vi "auto_transfer_output_dimension_withburnin.vi"() -> ()   [LabVIEW 2018]
panel:
  in  "Thickness (nm)":string
  in  "Dimension(No.:1-8)":fxp<+,8,8>=1.0 caption="Dimension"
  in  "Email on completion?":bool
  in  "Email recipient":string="rgiri@uw.edu"
  in  "Subject":string="OECT Scans Done"
  in  "Message":string="Hi Raj"
  out "Current Scan #":dbl
  out "Current V_G":dbl
  in  "Transfer Curve Controls":T1={"V_G Start"=-0.85, "V_G Finish"=0.0, "V_G Step Size"=0.025, "Software Averages"=5, "Delay between \naverages (ms)"=200.0, "Preread delay (ms)"=5000.0, "First bias settle (ms)"=2000.0, "V_DS"=-0.6, "Current Compliance\nLimit 237 (A)"=0.1, "Keithley 237 GPIB address"="17", "Current Compliance\nLimit (A) Ke2400"=1.0, "VISA resource name "="GPIB0::24::INSTR", "Number of Transfer Curves"=1.0, "Voltage Compliance Limit 237 (V)"=10.0} {"Voltage Compliance Limit 237 (V)" format="%#.3f"; "Current Compliance\nLimit (A) Ke2400" format="%#.3e"; "Current Compliance\nLimit 237 (A)" format="%#.3f"; "V_DS" format="%#_13g"; "First bias settle (ms)" format="%#.2f"; "Preread delay (ms)" format="%.2f"; "Delay between \naverages (ms)" format="%#.3f"; "V_G Step Size" format="%#.3g"; "V_G Finish" format="%#.3g"; "V_G Start" format="%#.3g"}
  in  "Output Curve Controls":T2={"V_DS Start"=-0.7, "V_DS Finish"=0.0, "V_DS Step Size"=0.1, "Software Averages"=5, "Delay between \naverages (ms)"=200.0, "Preread delay (ms)"=5000.0, "First bias settle (ms)"=2000.0, "Current Compliance\nLimit 237 (A)"=0.1, "Keithley 237 GPIB address"="17", "Current Compliance\nLimit (A) Ke2400"=1.0, "VISA resource name "="GPIB0::24::INSTR", "Voltage Compliance Limit 237 (V)"=10.0, "V_G Array"=[-0.5, -0.8]} {"Voltage Compliance Limit 237 (V)" format="%#.3f"; "Current Compliance\nLimit (A) Ke2400" format="%#.3e"; "Current Compliance\nLimit 237 (A)" format="%#.3f"; "First bias settle (ms)" format="%#.2f"; "Preread delay (ms)" format="%.2f"; "Delay between \naverages (ms)" format="%#.3f"; "V_DS Step Size" format="%#.3g"; "V_DS Finish" format="%#.3g"; "V_DS Start" format="%#.3g"}
  # "Output Curve Display"
  # "Transfer Curve Display"
  # "Scan Settings"
  # "Keithley 237 (V_DS) Settings"
  # "Keithley 2400 (V_G) Settings"
  # "Scan Settings"
  # "Keithley 237 (V_DS) Settings"
  # "Keithley 2400 (V_G) Settings"
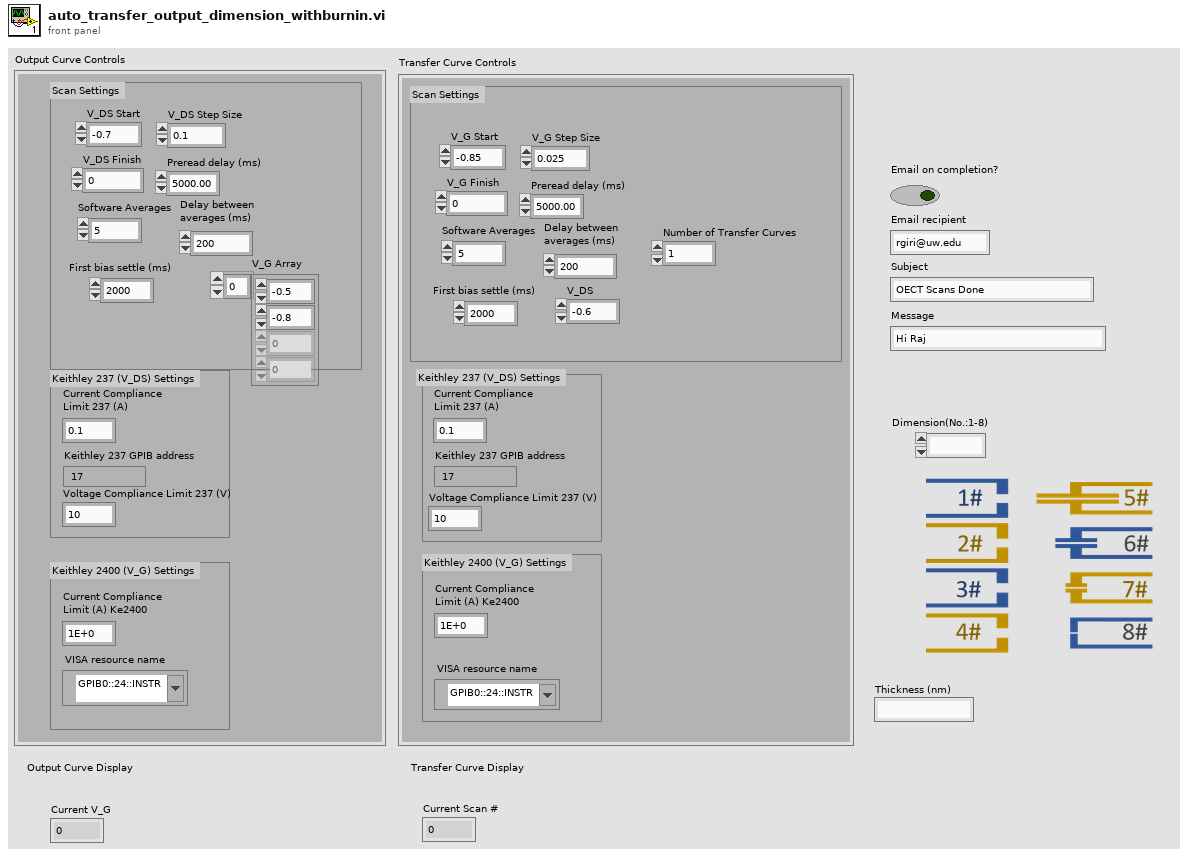
[diagram p1: front panel]
types:
  T1 = cluster{"V_G Start":dbl, "V_G Finish":dbl, "V_G Step Size":dbl, "Software Averages":i16, "Delay between \naverages (ms)":dbl, "Preread delay (ms)":dbl, "First bias settle (ms)":dbl, "V_DS":dbl, "Current Compliance\nLimit 237 (A)":dbl, "Keithley 237 GPIB address":string, "Current Compliance\nLimit (A) Ke2400":dbl, "VISA resource name ":refnum<visa-resource-name>, "Number of Transfer Curves":dbl, "Voltage Compliance Limit 237 (V)":dbl}
  T2 = cluster{"V_DS Start":dbl, "V_DS Finish":dbl, "V_DS Step Size":dbl, "Software Averages":i16, "Delay between \naverages (ms)":dbl, "Preread delay (ms)":dbl, "First bias settle (ms)":dbl, "Current Compliance\nLimit 237 (A)":dbl, "Keithley 237 GPIB address":string, "Current Compliance\nLimit (A) Ke2400":dbl, "VISA resource name ":refnum<visa-resource-name>, "Voltage Compliance Limit 237 (V)":dbl, "V_G Array":dbl[]}
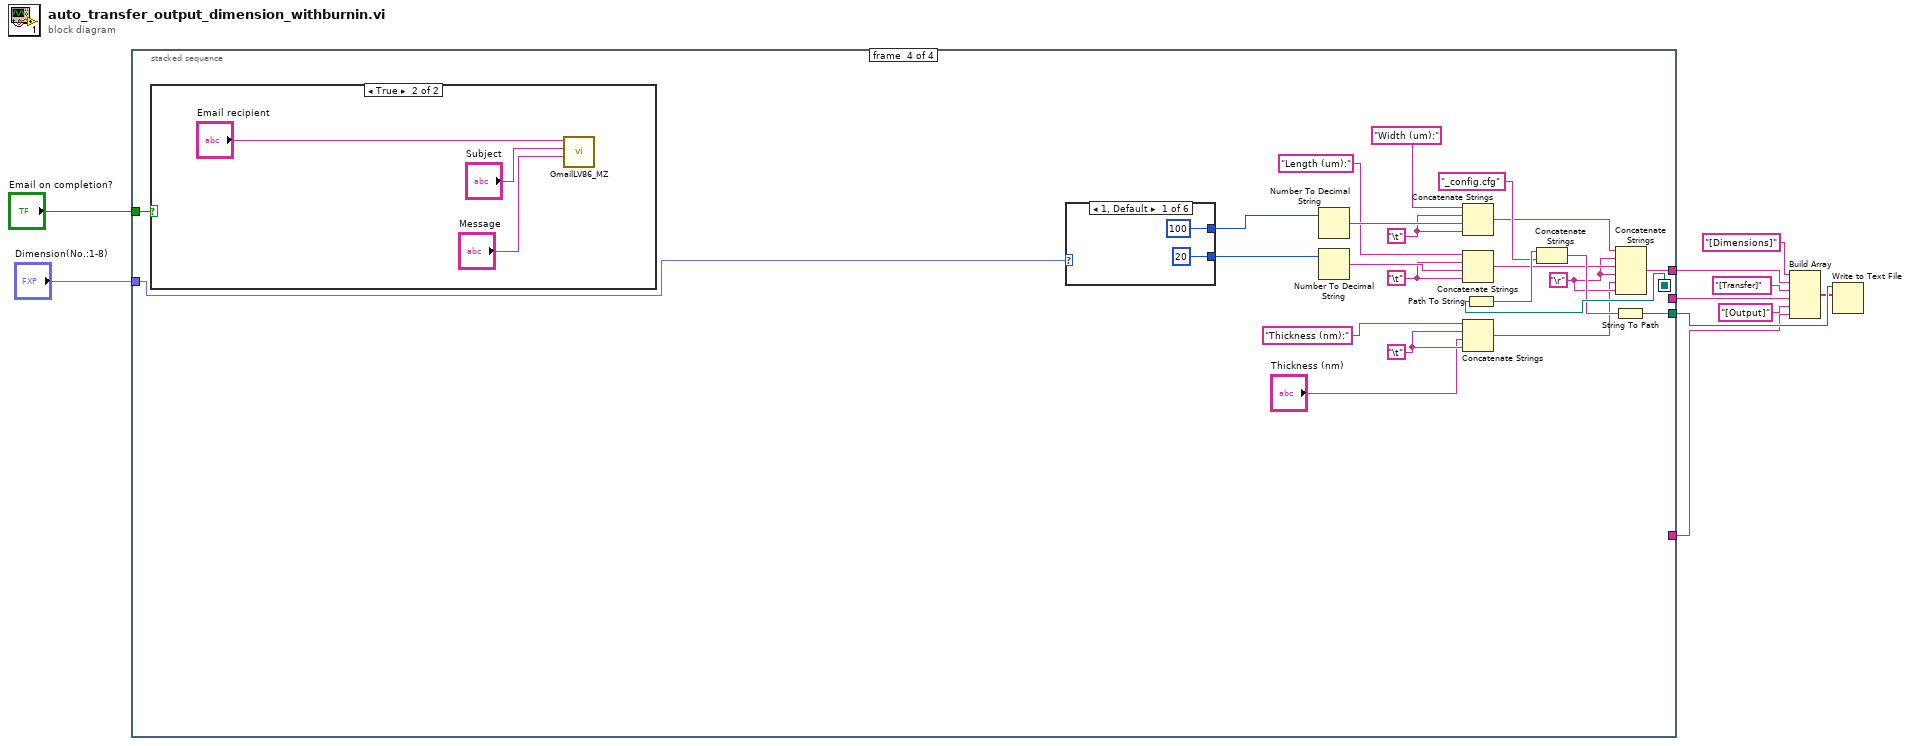
[diagram p0: block diagram]
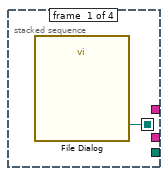
[diagram p2: hidden frame]
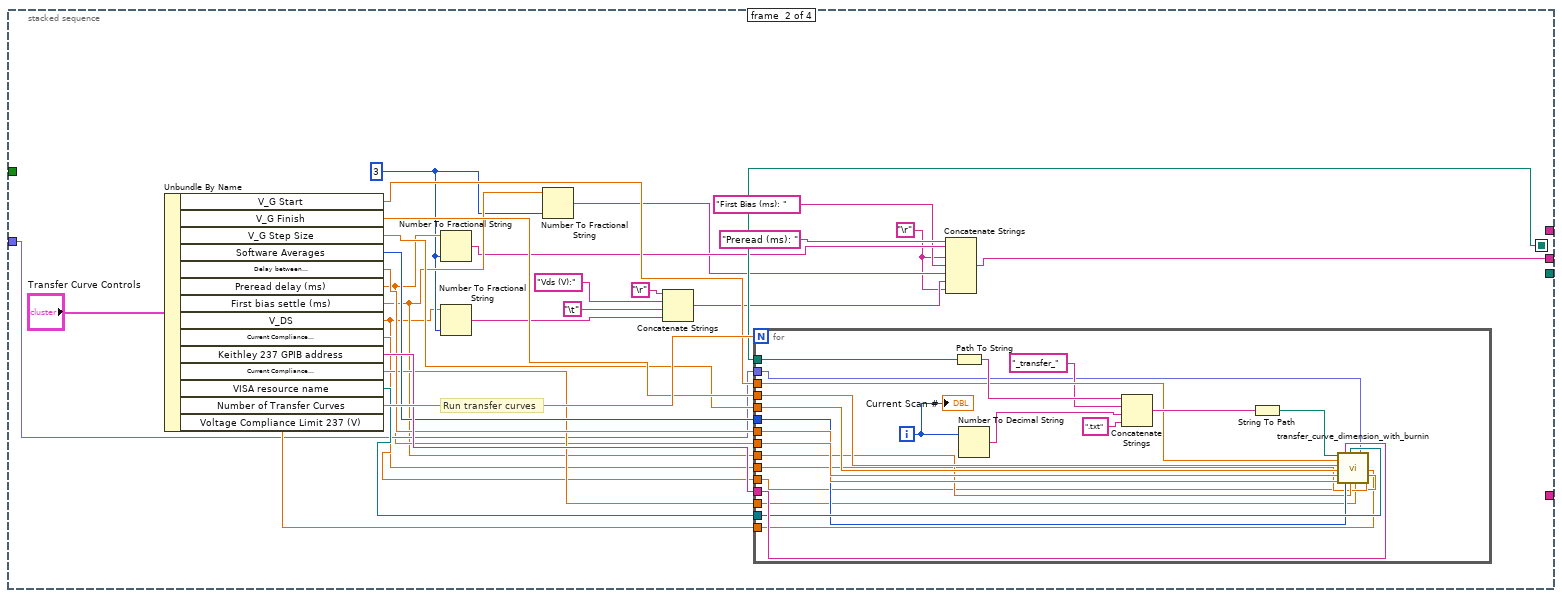
[diagram p3: hidden frame]
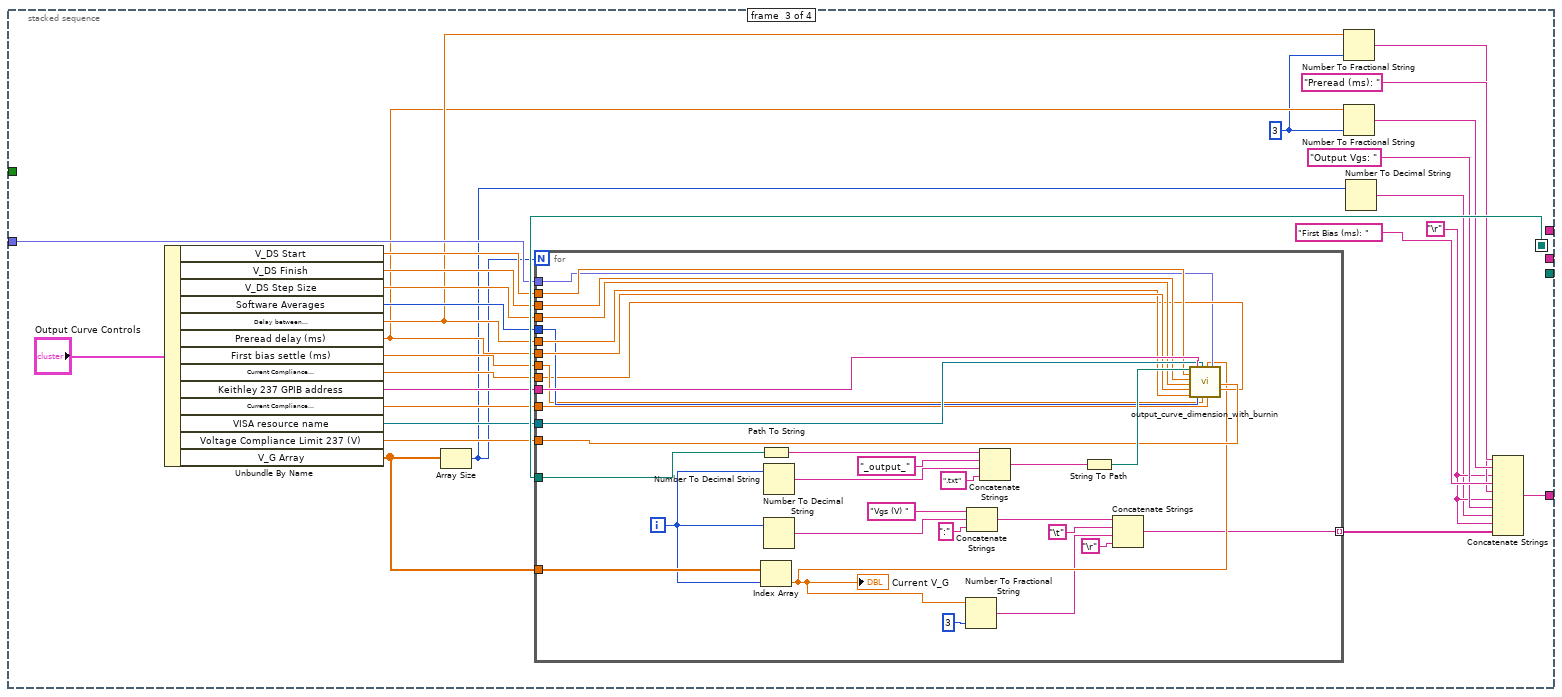
[diagram p4: hidden frame]
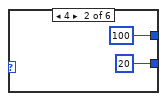
[diagram p5: hidden frame]
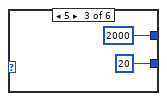
[diagram p6: hidden frame]
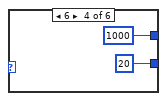
[diagram p7: hidden frame]
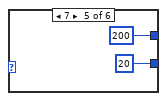
[diagram p8: hidden frame]
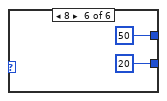
[diagram p9: hidden frame]
diagram:
  n1 = stacked-sequence {
    seq-local: [w11 _ _ _] -> [_ w38 w88 w143]
    tunnel: "Email on completion?" -> [_ _ _ w144]
    tunnel: "Dimension(No.:1-8)" -> [_ w27 w77 w139]
    tunnel: [_ w20 _ _] -> w5
    tunnel: [_ _ w69 _] -> w4
    tunnel: [_ _ _ w130] -> w8
    tunnel: [_ _ _ w127] -> w6
    frame #0 {
      n2 = call "File Dialog"() -> ("selected path"=w11:path)  [unwired: 12 in, 3 out]
    }
    frame #1 {
      w18 = 3
      w12 = "\r"
      # "Run transfer curves"
      n3 = Unbundle By Name("Transfer Curve Controls") -> ("V_G Start"=w35:dbl, "V_G Finish"=w34:dbl, "V_G Step Size"=w33:dbl, "Software Averages"=w31:i16, "Delay between \naverages (ms)"=w32:dbl, "Preread delay (ms)"=w26:dbl, "First bias settle (ms)"=w25:dbl, "V_DS"=w17:dbl, "Current Compliance\nLimit 237 (A)"=w29:dbl, "Keithley 237 GPIB address"=w37:string, "Current Compliance\nLimit (A) Ke2400"=w30:dbl, "VISA resource name"=w36:refnum<visa-resource-name>, "Number of Transfer Curves"=w39:dbl, "Voltage Compliance Limit 237 (V)"=w28:dbl)
      n4 = Number To Fractional String(number=w26, precision (6)=w18) -> (F-format string=w23:string)  [unwired: 2 in]
      n5 = Number To Fractional String(number=w17, precision (6)=w18) -> (F-format string=w15:string)  [unwired: 2 in]
      n6 = Number To Fractional String(number=w25, precision (6)=w18) -> (F-format string=w21:string)  [unwired: 2 in]
      n7 = Concatenate Strings("\r", "Vds (V):", "\t", w15) -> (w14:string)
      n8 = for {
        N: w39 -> [_]
        tunnel: w38 -> [w62]
        tunnel: w37 -> [w58]
        tunnel: w36 -> [w57]
        tunnel: w35 -> [w56]
        tunnel: w34 -> [w55]
        tunnel: w33 -> [w54]
        tunnel: w26 -> [w53]
        tunnel: w32 -> [w52]
        tunnel: w31 -> [w51]
        tunnel: w25 -> [w50]
        tunnel: w17 -> [w49]
        tunnel: w30 -> [w48]
        tunnel: w29 -> [w47]
        tunnel: w28 -> [w46]
        tunnel: w27 -> [w41]
        i -> [w42]
        n9 = Path To String(path=w62) -> (string=w61:string)
        n10 = Number To Decimal String(number=w42) -> (decimal integer string=w44:string)  [unwired: 1 in]
        n11 = Concatenate Strings(w61, "_transfer_", w44, ".txt") -> (w60:string)
        n12 = String To Path(string=w60) -> (path=w59:path)
        n13 = call "transfer_curve_dimension_with_burnin.vi"("File Path"=w59, "V_G Start"=w56, "V_G Finish"=w55, "V_G Step Size"=w54, "Preread delay (ms)"=w53, "Delay between \naverages (ms)"=w52, "Keithley 237 GPIB address"=w58, "Software Averages"=w51, "VISA resource name"=w57, "First bias settle (ms)"=w50, "Current Compliance\nLimit (A) Ke2400"=w48, "Dimension(No.:1-8)"=w41, "Voltage Compliance Limit 237 (V)"=w46, "Current Compliance\nLimit 237 (A)"=w47, "V_DS"=w49) -> ()  [unwired: 5 in]
        "Current Scan #" <- w42
      }
      n14 = Concatenate Strings("Preread (ms): ", w23, w12, "First Bias (ms): ", w21, w14, w12) -> (w20:string)
    }
    frame #2 {
      w65 = "\r"
      w66 = 3
      n15 = Unbundle By Name("Output Curve Controls") -> ("V_DS Start"=w85:dbl, "V_DS Finish"=w84:dbl, "V_DS Step Size"=w83:dbl, "Software Averages"=w82:i16, "Delay between \naverages (ms)"=w76:dbl, "Preread delay (ms)"=w75:dbl, "First bias settle (ms)"=w81:dbl, "Current Compliance\nLimit 237 (A)"=w78:dbl, "Keithley 237 GPIB address"=w87:string, "Current Compliance\nLimit (A) Ke2400"=w80:dbl, "VISA resource name"=w86:refnum<visa-resource-name>, "Voltage Compliance Limit 237 (V)"=w79:dbl, "V_G Array"=w74:dbl[])
      n16 = Array Size(array=w74) -> (size(s)=w64:i32)
      n17 = for {
        N: w64 -> [_]
        tunnel: w74 -> [w121]
        tunnel: w88 -> [w120]
        tunnel: w87 -> [w114]
        tunnel: w86 -> [w113]
        tunnel: w85 -> [w111]
        tunnel: w84 -> [w110]
        tunnel: w83 -> [w109]
        tunnel: w75 -> [w108]
        tunnel: w76 -> [w107]
        tunnel: w82 -> [w106]
        tunnel: w81 -> [w105]
        tunnel: w80 -> [w104]
        tunnel: w79 -> [w103]
        tunnel: w78 -> [w102]
        tunnel: w77 -> [w101]
        tunnel: [w97] -> w67 mode=indexing
        i -> [w94]
        n18 = Path To String(path=w120) -> (string=w119:string)
        n19 = Index Array(array=w121, index=w94) -> (element=w100:dbl)
        "Current V_G" <- w100
        n20 = Number To Decimal String(number=w94) -> (decimal integer string=w117:string)  [unwired: 1 in]
        n21 = Number To Decimal String(number=w94) -> (decimal integer string=w91:string)  [unwired: 1 in]
        n22 = Number To Fractional String(number=w100, precision (6)=3) -> (F-format string=w99:string)  [unwired: 2 in]
        n23 = Concatenate Strings("Vgs (V) ", w91, ":") -> (w92:string)
        n24 = Concatenate Strings(w119, "_output_", w117, ".txt") -> (w115:string)
        n25 = String To Path(string=w115) -> (path=w112:path)
        n26 = Concatenate Strings(w92, "\t", w99, "\r") -> (w97:string)
        n27 = call "output_curve_dimension_with_burnin.vi"("File Path"=w112, "V_DS Start"=w111, "V_DS Finish"=w110, "V_DS Step Size"=w109, "Preread delay (ms)"=w108, "Delay between \naverages (ms)"=w107, "Keithley 237 GPIB address"=w114, "Software Averages"=w106, "VISA resource name"=w113, "First bias settle (ms)"=w105, "V_G"=w100, "Current Compliance\nLimit (A) Ke2400"=w104, "Dimension(No.:1-8)"=w101, "Voltage Compliance Limit 237 (V)"=w103, "Current Compliance\nLimit 237 (A)"=w102) -> ()  [unwired: 5 in]
      }
      n28 = Number To Fractional String(number=w76, precision (6)=w66) -> (F-format string=w70:string)  [unwired: 2 in]
      n29 = Number To Fractional String(number=w75, precision (6)=w66) -> (F-format string=w72:string)  [unwired: 2 in]
      n30 = Number To Decimal String(number=w64) -> (decimal integer string=w63:string)  [unwired: 1 in]
      n31 = Concatenate Strings("Preread (ms): ", w72, w65, "First Bias (ms): ", w70, w65, "Output Vgs: ", w63, w65, w67) -> (w69:string)
    }
    frame #3 {
      w123 = "\t"
      w126 = "\r"
      w132 = "\t"
      w136 = "\t"
      n32 = case shown="True" w144 {
        frame False {
        }
        frame True {
          n33 = call "GmailLV86_MZ.vi"("Body"="Message", "Subject"="Subject", "Recipient's Email Address"="Email recipient") -> ()  [unwired: 7 in]
        }
      }
      n34 = case shown="1, Default" w139 {
        tunnel: [100 100 2000 1000 200 50] -> w135
        tunnel: [20 20 20 20 20 20] -> w131
        frame 1, Default {
        }
        frame 4 {
        }
        frame 5 {
        }
        frame 6 {
        }
        frame 7 {
        }
        frame 8 {
        }
      }
      n35 = Number To Decimal String(number=w135) -> (decimal integer string=w138:string)  [unwired: 1 in]
      n36 = Number To Decimal String(number=w131) -> (decimal integer string=w134:string)  [unwired: 1 in]
      n37 = Concatenate Strings("Width (um):", w136, w138, w136) -> (w129:string)
      n38 = Concatenate Strings("Length (um):", w132, w134, w132) -> (w128:string)
      n39 = Concatenate Strings("Thickness (nm):", w123, "Thickness (nm)", w123) -> (w125:string)
      n40 = Path To String(path=w143) -> (string=w142:string)
      n41 = Concatenate Strings(w142, "_config.cfg") -> (w140:string)
      n42 = String To Path(string=w140) -> (path=w130:path)
      n43 = Concatenate Strings(w129, w126, w128, w126, w125, w126) -> (w127:string)
    }
  }
  n44 = Build Array("[Dimensions]", w6, "[Transfer]", w5, "[Output]", w4) -> (w7:string[])
  n45 = Write to Text File(file (use dialog)=w8, text=w7) -> ()  [unwired: 2 in, 3 out]
